vi "GetPersistentConfiguration.vi"(8 "ErrorIn":errorcluster, 9 "DataIn":variant, 11 "ReferenceIn":refnum<class "DemoApplication.lvclass">) -> (0 "ErrorOut":errorcluster, 1 "DataOut":variant, 3 "ReferenceOut":refnum<class "DemoApplication.lvclass">)   [LabVIEW 2021, in "DemoApplication.lvclass"]
uses:
  DemoApplication.lvclass
  .Externals/Library_TAF_ApplicationFramework/MasterGUI/MasterGUI.lvclass
  DemoApplication.lvclass/DemoApplication.ctl
  C:/Localdata/Projects/TriekselSoft/TriekselsoftApplicationFramework/Source/.Externals/Library_TAF_ApplicationFramework/MasterGUI/MasterGUI.lvclass
  C:/Localdata/Projects/TriekselSoft/TriekselsoftApplicationFramework/Source/.Externals/Library_TAF_ApplicationFramework/TAFBaseGUI/TAFBaseGUI.lvclass
  C:/Localdata/Projects/TriekselSoft/TriekselsoftApplicationFramework/Source/.Externals/Interface_TAF_AutorizationUpdated/IAuthorizationUpdated/IAuthorizationUpdated.lvclass
  C:/Localdata/Projects/TriekselSoft/TriekselsoftApplicationFramework/Source/IInterface/IInterface.lvclass
  C:/Localdata/Projects/TriekselSoft/TriekselsoftApplicationFramework/Source/.Externals/Interface_UserInterface_IDockGUI/IDockGUI/IDockGUI.lvclass
  C:/Localdata/Projects/TriekselSoft/TriekselsoftApplicationFramework/Source/.Externals/Interface_UserInterface_IFrontPanel/IFrontPanel/IFrontPanel.lvclass
  C:/Localdata/Projects/TriekselSoft/TriekselsoftApplicationFramework/Source/.Externals/Interface_TAF_ITAFGUIActions/ITAFGUIActions/ITAFGUIActions.lvclass
  C:/Localdata/Projects/TriekselSoft/TriekselsoftApplicationFramework/Source/.Externals/Interface_Object_ICreateDestroy/ICreateDestroy/ICreateDestroy.lvclass
  C:/Localdata/Projects/TriekselSoft/TriekselsoftApplicationFramework/Source/.Externals/Interface_Object_IPersistentData/IPersistentData/IPersistentData.lvclass
  C:/Localdata/Projects/TriekselSoft/TriekselsoftApplicationFramework/Source/.Externals/Interface_TAF_ITAFObject/ITAFObject/ITAFObject.lvclass
  C:/Localdata/Projects/TriekselSoft/TriekselsoftApplicationFramework/Source/DemoApplication/DemoApplication.lvclass
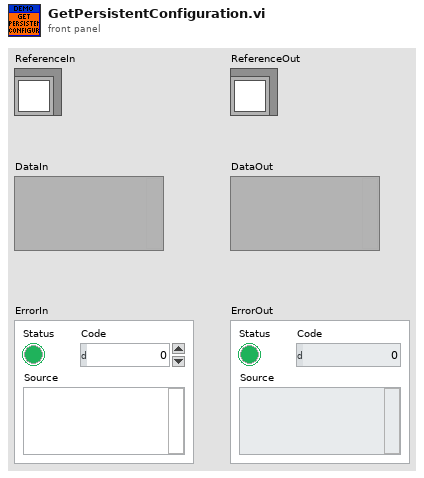
[diagram p1: front panel]
types:
  T1 = typedef "DemoApplication.lvclass/ObjectAttributes.ctl" = cluster{"Interfaces":cluster{"Authorizer":refnum<class "IAuthorization.lvclass">, "TextViewer":refnum<class "ITAFTextViewer.lvclass">, "ApplicationConfiguration":refnum<class "IApplicationConfiguration.lvclass">, "Tracer":refnum<class "IFrontPanel.lvclass">}, "Persistent":cluster{"MenuEnables":cluster{"MenuTag":string, "MenuExpression":string}[], "TextDockSubPanelName":string}}
  T2 = cluster{"MenuEnables":cluster{"MenuTag":string, "MenuExpression":string}[], "TextDockSubPanelName":string}
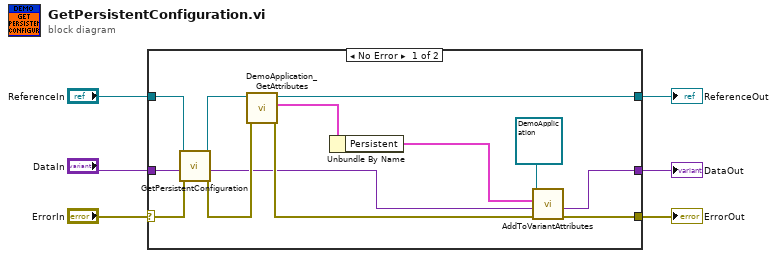
[diagram p0: block diagram]
diagram:
  n1 = case shown="No Error" "ErrorIn" {
    selector: "ErrorIn" -> [w19 w22]
    tunnel: [w17 w22] -> w5
    tunnel: [w14 w21] -> w3
    tunnel: "ReferenceIn" -> [w10 w21]
    tunnel: [w13 w20] -> w2
    tunnel: "DataIn" -> [w8 w20]
    frame No Error {
      n2 = call-parent "GetPersistentConfiguration.vi"("ErrorIn"=w19, "DataIn"=w8, "ReferenceIn"=w10) -> ("ErrorOut"=w16:errorcluster, "DataOut"=w7:variant, "ReferenceOut"=w9:refnum<class "DemoApplication.lvclass">)  [unwired: 6 in]
      n3 = call "DemoApplication_GetAttributes.vi"("ErrorIn"=w16, "ReferenceIn"=w9) -> ("ErrorOut"=w18:errorcluster, "Data"=w15:T1, "ReferenceOut"=w14:refnum<class "DemoApplication.lvclass">)  [unwired: 6 in, 1 out]
      n4 = Unbundle By Name(w15) -> ("Persistent"=w12:T2)
      n5 = call "AddToVariantAttributes.vi"("ErrorIn"=w18, "DataInIn"=w7, "PersistentData"=w12, "Object"=refnum<class "DemoApplication.lvclass"> refnum ("VerticalButtonBar")) -> ("ErrorOut"=w17:errorcluster, "DataInOut"=w13:variant)  [unwired: 6 in]
    }
    frame Error {
    }
  }
  "ErrorOut" <- w5
  "ReferenceOut" <- w3
  "DataOut" <- w2
